vi "Write Ref TC and Order.vi"(8 "error in (no error)":errorcluster, 9 "order":i32, 10 "TC (s)":dbl, 11 "LockinDAQ":refnum<class "LockinDAQ.lvclass">) -> (0 "error out":errorcluster, 3 "LockinDAQ out":refnum<class "LockinDAQ.lvclass">)   [LabVIEW 2016, in "LockinDAQ.lvclass"]
uses:
  LockinDAQ.lvclass
  LockinDAQ.lvclass/LockinDAQ.ctl
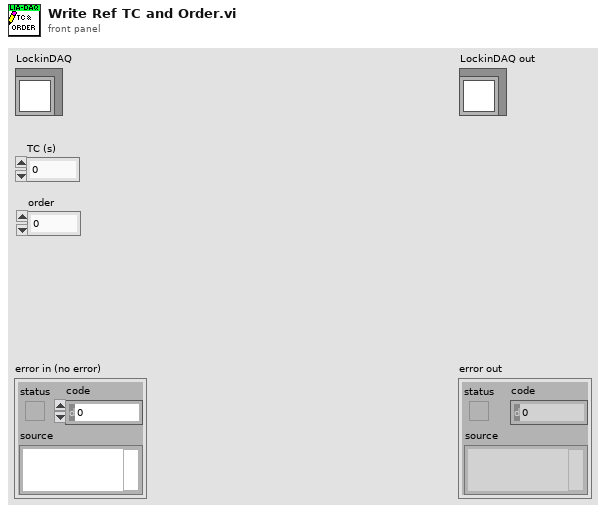
[diagram p1: front panel]
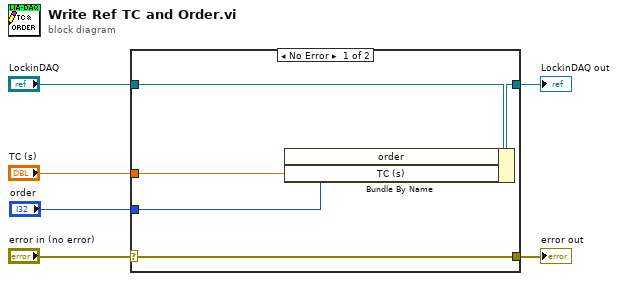
[diagram p0: block diagram]
diagram:
  n1 = case shown="No Error" "error in (no error)" {
    selector: "error in (no error)" -> [w11 w12]
    tunnel: [w11 w12] -> w5
    tunnel: [w9 w13] -> w3
    tunnel: "LockinDAQ" -> [w10 w13]
    tunnel: "TC (s)" -> [w8 _]
    tunnel: "order" -> [w7 _]
    frame No Error {
      n2 = Bundle By Name(cluster=w10, "order"=w7, "TC (s)"=w8) -> (w9:refnum<class "LockinDAQ.lvclass">)
    }
    frame Error {
    }
  }
  "error out" <- w5
  "LockinDAQ out" <- w3
